vi "Send and Plot XYYY Data.vi"() -> ()   [LabVIEW 2020]
panel:
  out "error out":errorcluster
  in  "Y3 Units":string
  in  "Y3 Long Name":string
  in  "Y2 Units":string
  in  "Y2 Long Name":string
  in  "Y1 Units":string
  in  "Y1 Long Name":string
  in  "X Units":string
  in  "X Long Name":string
  in  "X Value":dbl
  in  "stop":bool
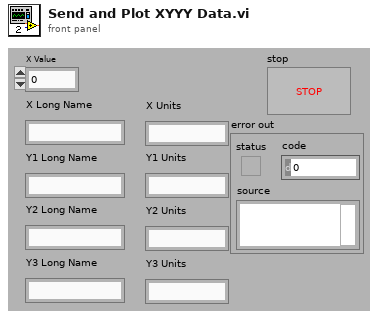
[diagram p1: front panel]
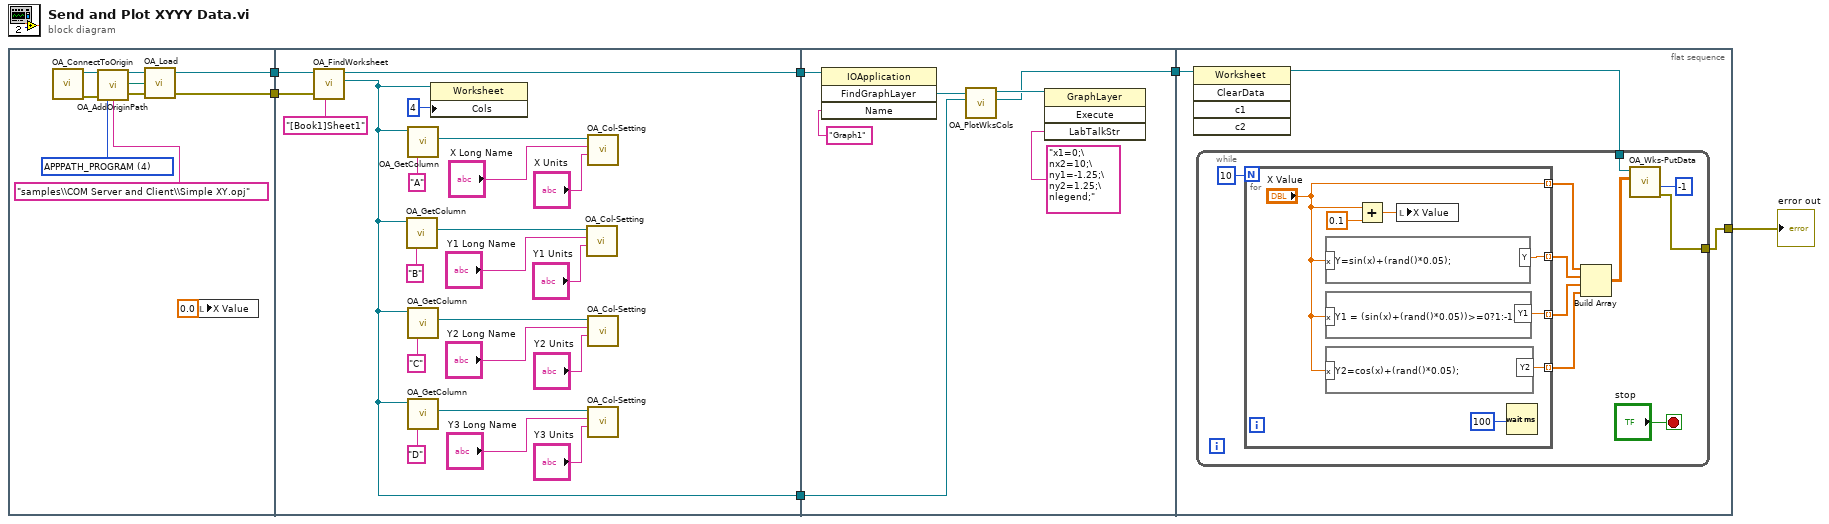
[diagram p0: block diagram]
diagram:
  n1 = flat-sequence {
    tunnel: [w8] -> w5
    tunnel: [w7] -> w4
    tunnel: w5 -> [w37]
    tunnel: w4 -> [w36]
    tunnel: [w17] -> w3
    tunnel: [w35] -> w2
    tunnel: [w39] -> w6
    tunnel: w3 -> [w42]
    tunnel: w2 -> [w44]
    tunnel: w6 -> [w48]
    tunnel: [w46] -> w1
    frame #0 {
      w14 = 4 items=["APPPATH_USER"=2, "APPPATH_GROUP"=3, "APPPATH_PROGRAM"=4] ("Type")
      n2 = call "OA_ConnectToOrigin.vi"() -> ("error out"=w9:errorcluster, "Origin.IOApplication"=w16:refnum<k7>)  [unwired: 8 in]
      n3 = call "OA_AddOriginPath.vi"("Origin.IOApplication"=w16, "error in (no error)"=w9, "Type"=w14, "Filename"="samples\\COM Server and Client\\Simple XY.opj" ("related path")) -> ("Origin.IOApplication"=w11:refnum<k7>, "path out"=w13:path, "error out"=w12:errorcluster)  [unwired: 9 in]
      n4 = call "OA_Load.vi"("error in (no error)"=w12, "Path"=w13, "Origin.IOApplication"=w11) -> ("error out"=w8:errorcluster, "Origin.IOApplication"=w7:refnum<k7>)  [unwired: 1 out]
      n5 = local write "X Value"(0.0 ("X Value")) -> ()
    }
    frame #1 {
      n6 = call "OA_FindWorksheet.vi"("Name"="[Book1]Sheet1", "error in (no error)"=w37, "Origin.IOApplication"=w36) -> ("Origin.Worksheet"=w17:refnum<k7>, "Origin.IOApplication"=w35:refnum<k7>)  [unwired: 6 in, 1 out]
      n7 = call "OA_GetColumn.vi"("Column Name/Index"="B" ("Name"), "Origin.Worksheet"=w17) -> ("Origin.Column"=w29:refnum<k7>)  [unwired: 7 in, 2 out]
      n8 = call "OA_GetColumn.vi"("Column Name/Index"="A" ("Name"), "Origin.Worksheet"=w17) -> ("Origin.Column"=w33:refnum<k7>)  [unwired: 7 in, 2 out]
      n9 = call "OA_GetColumn.vi"("Column Name/Index"="C" ("Name"), "Origin.Worksheet"=w17) -> ("Origin.Column"=w25:refnum<k7>)  [unwired: 7 in, 2 out]
      n10 = call "OA_GetColumn.vi"("Column Name/Index"="D" ("Name"), "Origin.Worksheet"=w17) -> ("Origin.Column"=w21:refnum<k7>)  [unwired: 7 in, 2 out]
      n11 = property class="Worksheet"(reference=w17, "Cols"=4) -> ()  [unwired: 1 in, 2 out]
      n12 = call "OA_Col-Setting.vi"("Origin.Column"=w29, "LongName"="Y1 Long Name", "Units"="Y1 Units") -> ()  [unwired: 4 in, 2 out]
      n13 = call "OA_Col-Setting.vi"("Origin.Column"=w33, "LongName"="X Long Name", "Units"="X Units") -> ()  [unwired: 4 in, 2 out]
      n14 = call "OA_Col-Setting.vi"("Origin.Column"=w25, "LongName"="Y2 Long Name", "Units"="Y2 Units") -> ()  [unwired: 4 in, 2 out]
      n15 = call "OA_Col-Setting.vi"("Origin.Column"=w21, "LongName"="Y3 Long Name", "Units"="Y3 Units") -> ()  [unwired: 4 in, 2 out]
    }
    frame #2 {
      n16 = invoke class="IOApplication" method="FindGraphLayer"(reference=w44, "Name"="Graph1" ("related path")) -> ("FindGraphLayer"=w41:refnum<k7>)  [unwired: 2 in, 3 out]
      n17 = call "OA_PlotWksCols.vi"("Origin.Worksheet in"=w42, "Origin.GraphLayer in"=w41) -> ("Origin.Worksheet Out"=w39:refnum<k7>, "Origin.GraphLayer Out"=w40:refnum<k7>)  [unwired: 6 in, 2 out]
      n18 = invoke class="GraphLayer" method="Execute"(reference=w40, "LabTalkStr"="x1=0;\nx2=10;\ny1=-1.25;\ny2=1.25;\nlegend;") -> ()  [unwired: 2 in, 4 out]
    }
    frame #3 {
      n19 = invoke class="Worksheet" method="ClearData"(reference=w48) -> (reference out=w47:refnum<k7>)  [unwired: 4 in, 4 out]
      n20 = while {
        tunnel: w47 -> [w55]
        tunnel: [w49] -> w46
        stop <- "stop" stop-if-true
        n21 = for {
          N: 10 -> [_]
          tunnel: [w65] -> w52 mode=indexing
          tunnel: ["X Value"] -> w51 mode=indexing
          tunnel: [w61] -> w53 mode=indexing
          tunnel: [w59] -> w54 mode=indexing
          n22 = formula code="Y=sin(x)+(rand()*0.05);"("x"="X Value") -> ("Y"=w65:dbl)
          n23 = formula code="Y1 = (sin(x)+(rand()*0.05))>=0?1:-1;"("x"="X Value") -> ("Y1"=w61:dbl)
          n24 = formula code="Y2=cos(x)+(rand()*0.05);"("x"="X Value") -> ("Y2"=w59:dbl)
          n25 = Add(x="X Value", y=0.1) -> (x+y=w62:dbl)
          n26 = local write "X Value"(w62) -> ()
          n27 = Wait (ms)(milliseconds to wait=u32 100) -> ()  [unwired: 1 out]
        }
        n28 = Build Array(w51, w52, w53, w54) -> (w50:dbl[][])
        n29 = call "OA_Wks-PutData.vi"("Row 1"=-1, "2d Data"=w50, "Origin.Worksheet"=w55) -> ("error out"=w49:errorcluster)  [unwired: 2 in, 2 out]
      }
    }
  }
  "error out" <- w1
